vi "Size.vi"(8 "error in (no error)":errorcluster, 11 "I32 Array in":refnum<class "I32 Array.lvclass">) -> (0 "error out":errorcluster, 2 "Size":i32, 3 "I32 Array out":refnum<class "I32 Array.lvclass">)   [LabVIEW 2020, in "Data.lvlib" / "I32 Array.lvclass"]
doc: "Return the size of the generic data element."
uses:
  I32 Array.lvclass
  I32 Array.lvclass/I32 Array.ctl
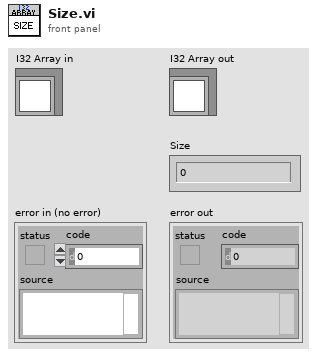
[diagram p1: front panel]
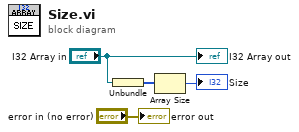
[diagram p0: block diagram]
diagram:
  n1 = Unbundle("I32 Array in") -> (w2:i32[])
  n2 = Array Size(array=w2) -> (size(s)=→"Size":i32)
  "error out" <- "error in (no error)"
  "I32 Array out" <- "I32 Array in"
